vi "난수발생.vi"() -> ()   [LabVIEW 2014]
panel:
  in  "경로":path
  in  "메뉴바/도구바":bool
  in  "정지":bool
  in  "난수발생":bool
  in  "가운데로":bool
  out "웨이브폼 차트":dbl(graph)
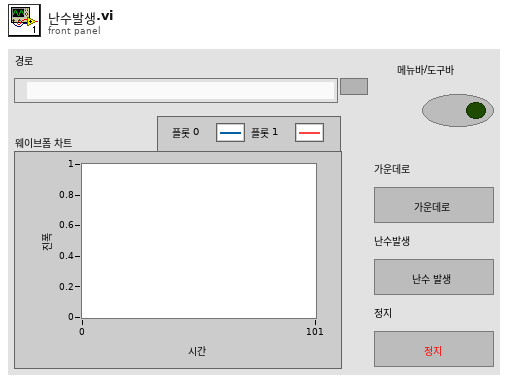
[diagram p1: front panel]
types:
  T1 = enum16{"Always On", "Always Off", "Off While Running"}
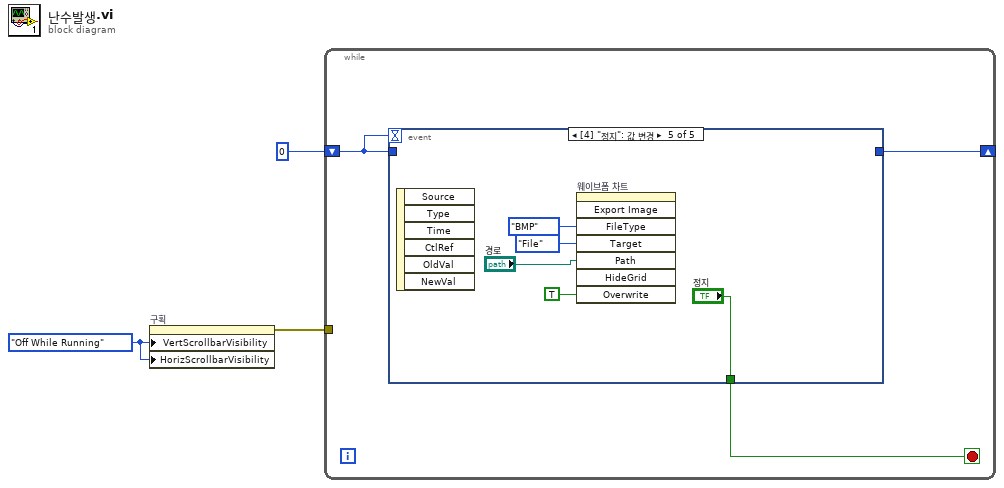
[diagram p0: block diagram]
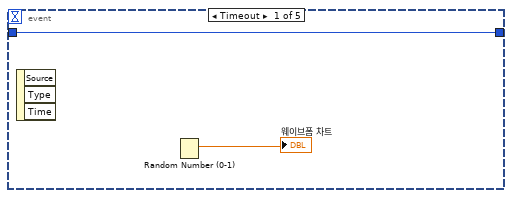
[diagram p2: hidden frame]
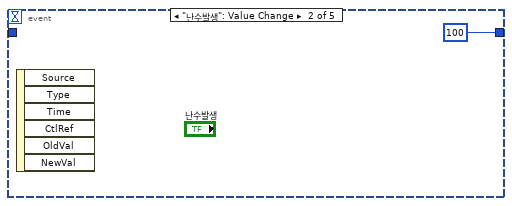
[diagram p3: hidden frame]
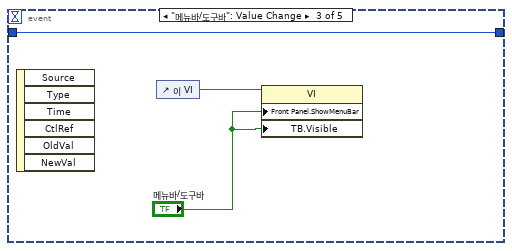
[diagram p4: hidden frame]
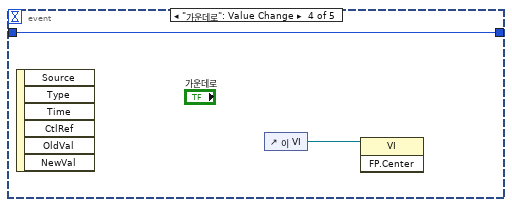
[diagram p5: hidden frame]
diagram:
  w2 = T1."Off While Running" ("수직 스크롤 막대 보이기")
  n1 = property on="구획" class="Pane"("VertScrollbarVisibility"=w2, "HorizScrollbarVisibility"=w2) -> (error out=w1:errorcluster)  [unwired: 2 in, 1 out]
  n2 = while {
    shift-right: [w5] -> _
    shift-left: 0 -> [w6]
    tunnel: w1 -> [_]
    stop <- w4 stop-if-true
    n3 = event shown="[4] \"정지\": 값 변경" {
      selector: _ -> [_ _ _ _ _]
      dyn-events: _ -> [_ _ _ _ _]
      timeout: w6 -> [_ _ _ _ _]
      tunnel: w6 -> [w8 _ w10 w13 _]
      tunnel: [w8 100 w10 w13 _] -> w5
      tunnel: [_ _ _ _ "정지"] -> w4
      event Timeout {
        n4 = event-data() -> ()  [unwired: 1 in, 3 out]
        n5 = Random Number (0-1)() -> (number: 0 to 1=→"웨이브폼 차트":dbl)
      }
      event "난수발생": Value Change {
        n6 = event-data() -> ()  [unwired: 1 in, 6 out]
      }
      event "메뉴바/도구바": Value Change {
        n7 = event-data() -> ()  [unwired: 1 in, 6 out]
        n8 = control-ref of="이 VI"() -> (w12:refnum<vi>)
        n9 = property class="VI"(reference=w12, "Front Panel.ShowMenuBar"="메뉴바/도구바", "TB.Visible"="메뉴바/도구바") -> ()  [unwired: 1 in, 2 out]
      }
      event "가운데로": Value Change {
        n10 = event-data() -> ()  [unwired: 1 in, 6 out]
        n11 = control-ref of="이 VI"() -> (w14:refnum<vi>)
        n12 = invoke class="VI" method="FP.Center"(reference=w14) -> ()  [unwired: 2 in, 3 out]
      }
      event "정지": Value Change {
        n13 = event-data() -> ()  [unwired: 1 in, 6 out]
        n14 = invoke on="웨이브폼 차트" class="WFChart (엄격한)" method="Export Image"("FileType"=enum32{"BMP", "EPS", "EMF", "PICT"}."BMP" ("파일 타입"), "Target"=enum32{"File", "Clipboard"}."File" ("타겟"), "Path"="경로", "Overwrite"=TRUE ("항상 덮어쓰기")) -> ()  [unwired: 4 in, 8 out]
      }
    }
  }
